vi "D_bank_Manual_Control_03.vi"(0 "SI804.lvclass in":refnum<class "SI804.lvclass">, 5 "3 JSD20 DT304\nXA01":dbl, 7 "3 JSD20 DT305\nXA01":dbl, 11 "error in":errorcluster) -> (4 "SI804.lvclass out":refnum<class "SI804.lvclass">, 6 "D-bk single in":dbl, 8 "D-bk single wdr":dbl, 15 "error out":errorcluster)   [LabVIEW 2022 SP3, in "SI804.lvclass"]
uses:
  SI804.lvclass
  SI804.lvclass/SI804.ctl
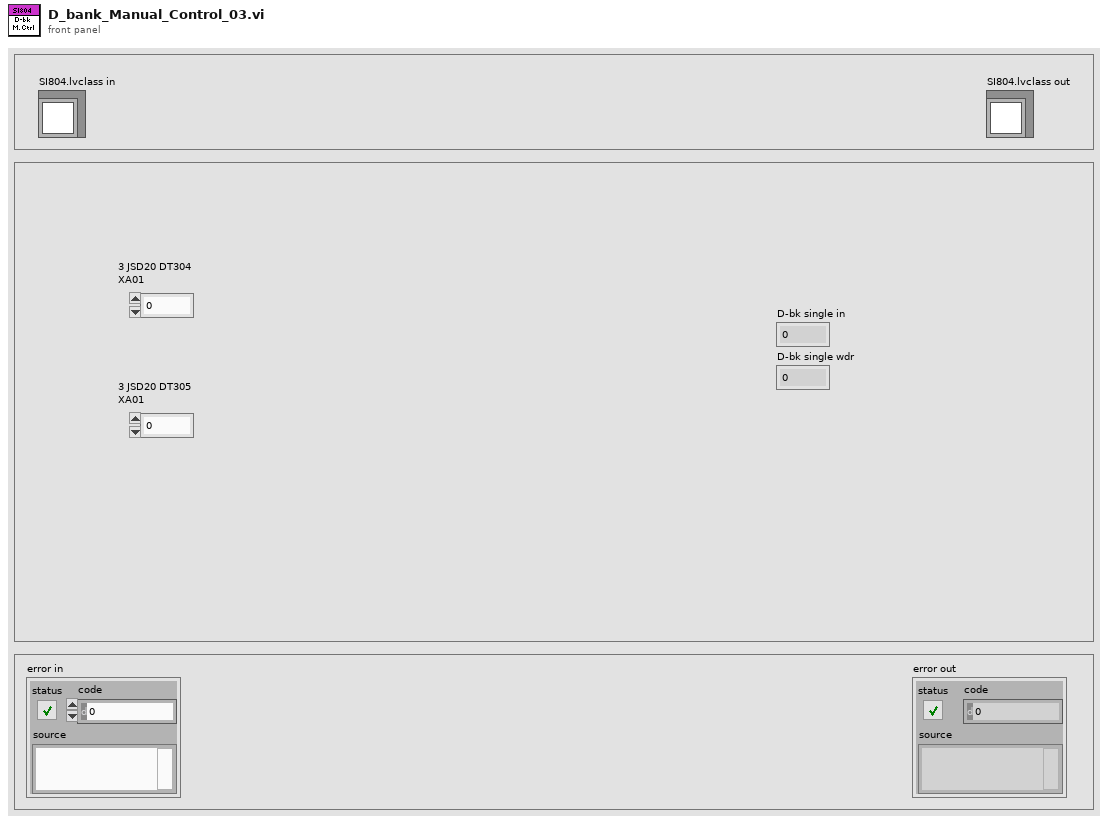
[diagram p1: front panel]
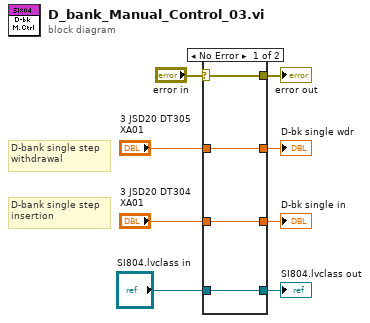
[diagram p0: block diagram]
diagram:
  # "D-bank single step\nwithdrawal"
  # "D-bank single step\ninsertion"
  n1 = case shown="No Error" "error in" {
    selector: "error in" -> [w9 w13]
    tunnel: "3 JSD20 DT304\nXA01" -> [w12 _]
    tunnel: "3 JSD20 DT305\nXA01" -> [w11 _]
    tunnel: "SI804.lvclass in" -> [w10 w14]
    tunnel: [w12 _] -> w3
    tunnel: [w11 _] -> w2
    tunnel: [w10 w14] -> w4
    tunnel: [w9 w13] -> w1
    frame No Error {
    }
    frame Error {
    }
  }
  "SI804.lvclass out" <- w4
  "D-bk single in" <- w3
  "D-bk single wdr" <- w2
  "error out" <- w1
